vi "parsing-demo.vi"() -> ()   [LabVIEW 2017]
panel:
  out "JSON string":string
  out "array":string[](array[string])
  in  "stack-conf":string
  in  "command":string="a\na\na\n"
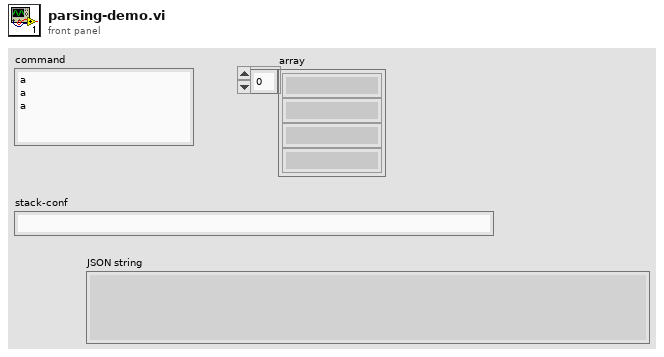
[diagram p1: front panel]
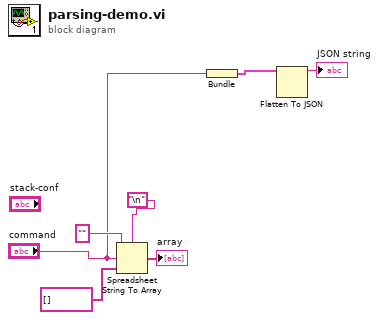
[diagram p0: block diagram]
diagram:
  n1 = Spreadsheet String To Array(delimiter (Tab)="\n", format string="", spreadsheet string="command", array type (2D Dbl)=string[] []) -> (array=→"array":string[])
  n2 = Bundle("command"="command") -> (w2:cluster{"command":string})  [unwired: 1 in]
  n3 = Flatten To JSON(anything=w2) -> (JSON string=→"JSON string":string)  [unwired: 2 in, 1 out]
